vi "Read Number.vi"(8 "error in (no error)":errorcluster, 11 "Simulado in":refnum<class "Simulado.lvclass">) -> (0 "error out":errorcluster, 2 "Number Read":string, 3 "Simulado out":refnum<class "Simulado.lvclass">)   [LabVIEW 2020, in "Simulado.lvclass"]
uses:
  Simulado.lvclass
  Simulado.lvclass/Simulado.ctl
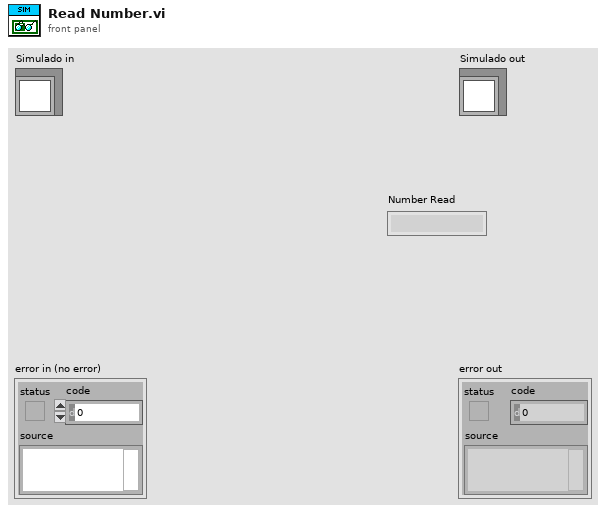
[diagram p1: front panel]
types:
  T1 = enum16{"Get Parameters", "Set Parameters", "Reset"}
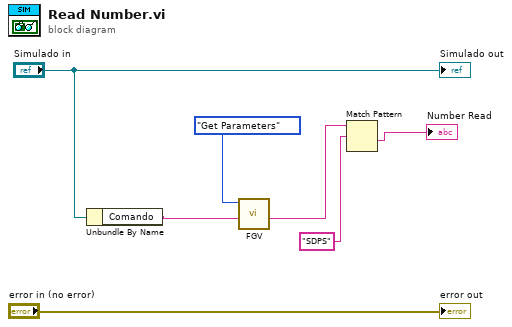
[diagram p0: block diagram]
diagram:
  n1 = Unbundle By Name("Simulado in") -> ("Comando"=w2:string)
  n2 = call "FGV.vi"("Comandos"=w2, "Función"=T1."Get Parameters") -> ("Respuesta"=w5:string)  [unwired: 9 in]
  n3 = Match Pattern(string=w5, regular expression="SDPS") -> (after substring=→"Number Read":string)  [unwired: 1 in, 3 out]
  "error out" <- "error in (no error)"
  "Simulado out" <- "Simulado in"
